vi "FormatDMAelement_6_elements.vi"(8 "valid in":bool, 10 "factor":u16, 11 "Data in":fxp<+/-,32,14>[](array[numeric])=[0.0, 0.0, 0.0, 0.0, 0.0, 0.0]) -> (0 "valid out":bool, 3 "Values":u64[](array[numeric]))   [LabVIEW 2018]
uses:
  <vilib>/rvi/FXPMathLib/FxpConvert/subVIs/nifxpmath_Convert_SimConfig.ctl
  <vilib>/fxp/LVFixedPointQuantizationPolicyTypeDef.ctl
  <vilib>/fxp/LVFixedPointOverflowPolicyTypeDef.ctl
  <vilib>/rvi/FXPMathLib/FxpConvert/simVIs/DllFxpConvertTemp_sub.vi
  <vilib>/rvi/FXPMathLib/FxpConvert/XNode/nifxpmath_Convert.xnode
  <vilib>/rvi/FXPMathLib/FxpInterpret/XNode/nifxpmath_Interpret.xnode
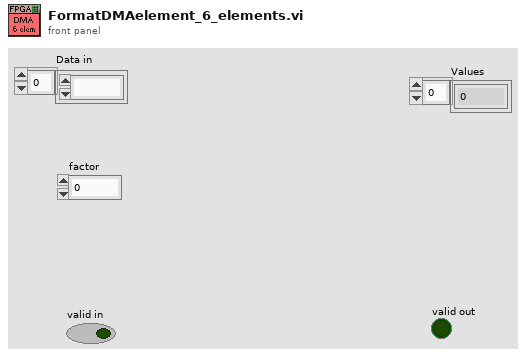
[diagram p1: front panel]
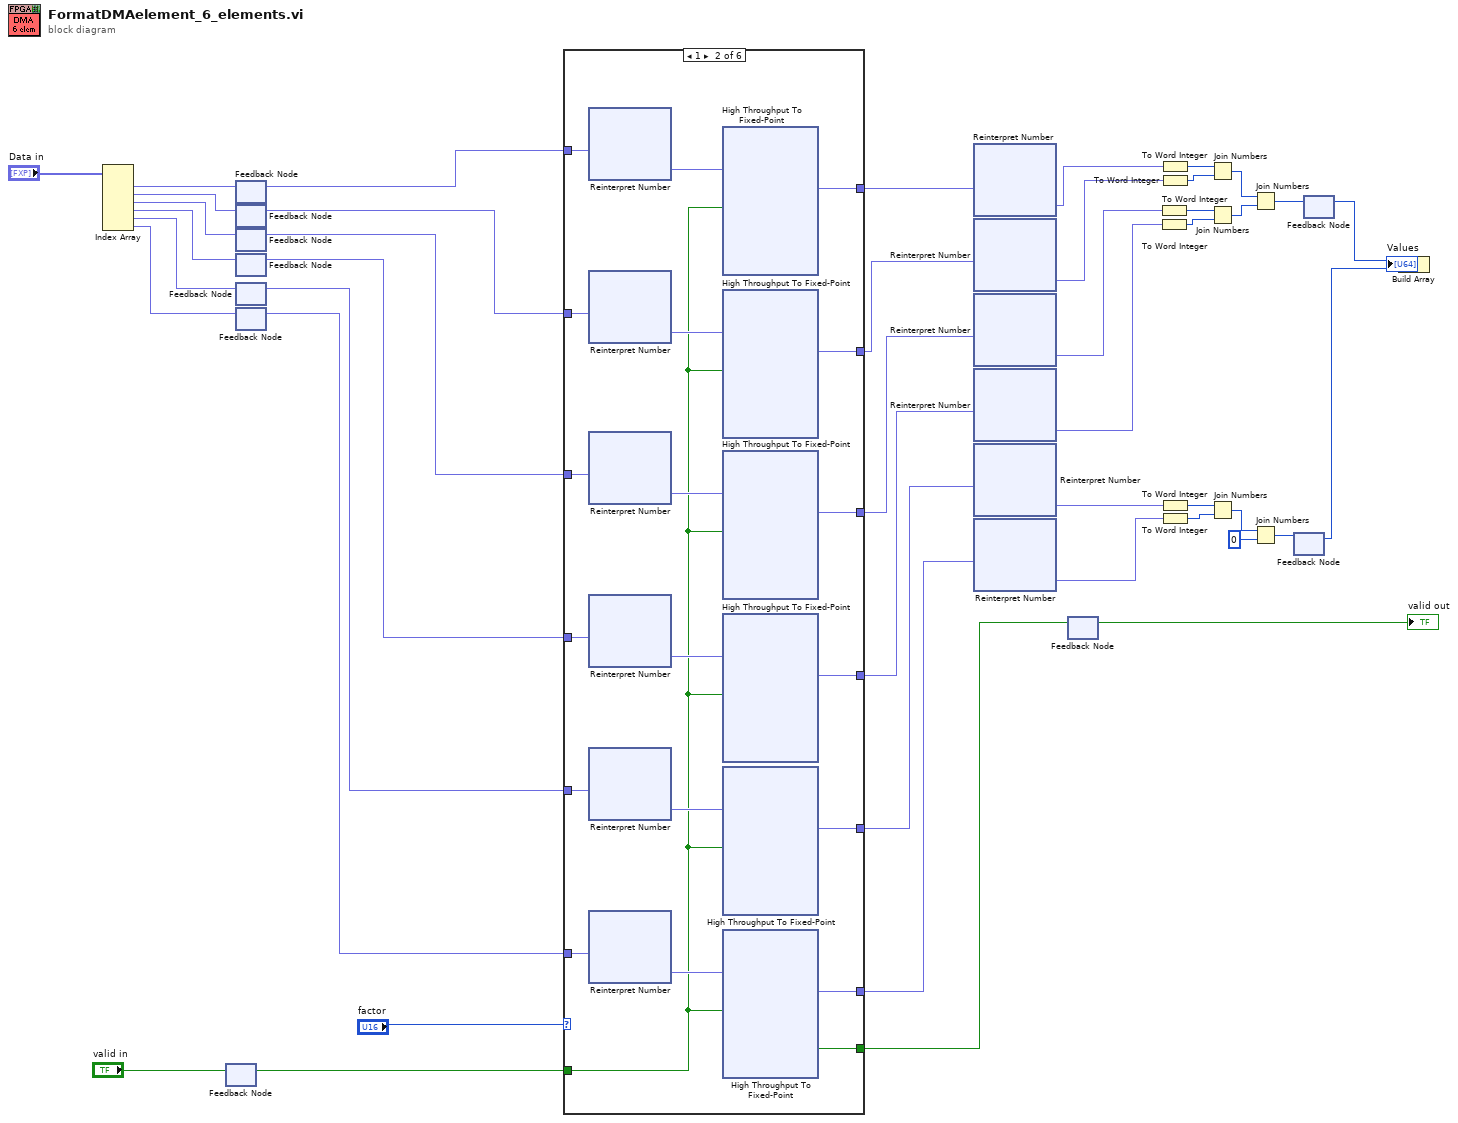
[diagram p0: block diagram]
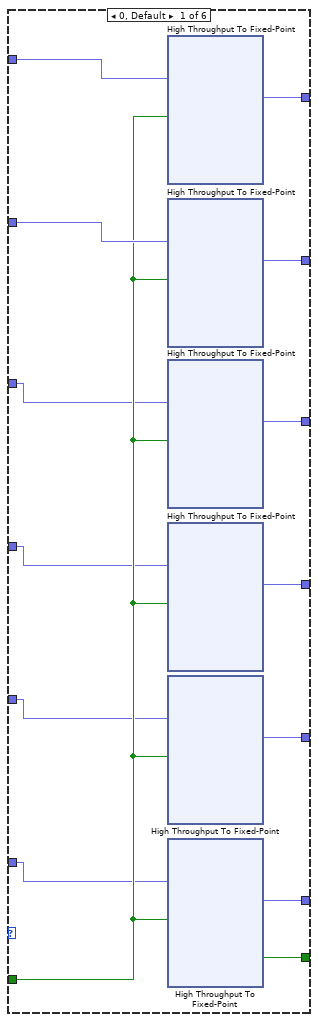
[diagram p2: hidden frame]
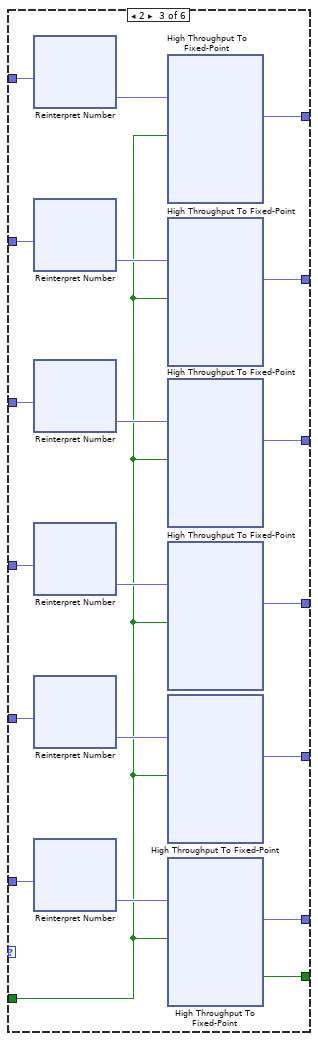
[diagram p3: hidden frame]
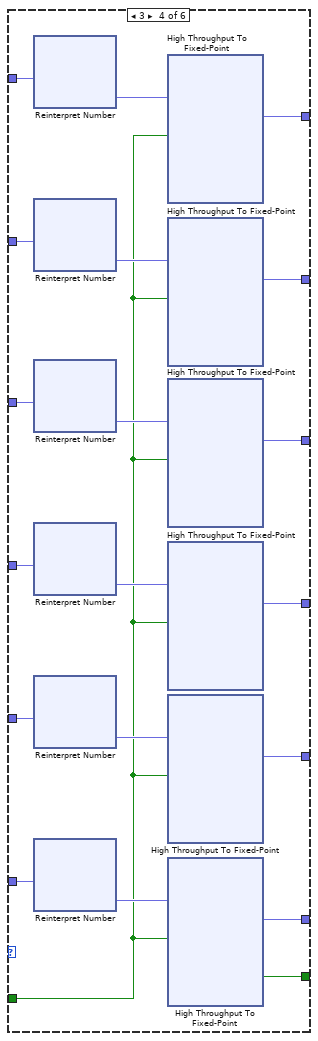
[diagram p4: hidden frame]
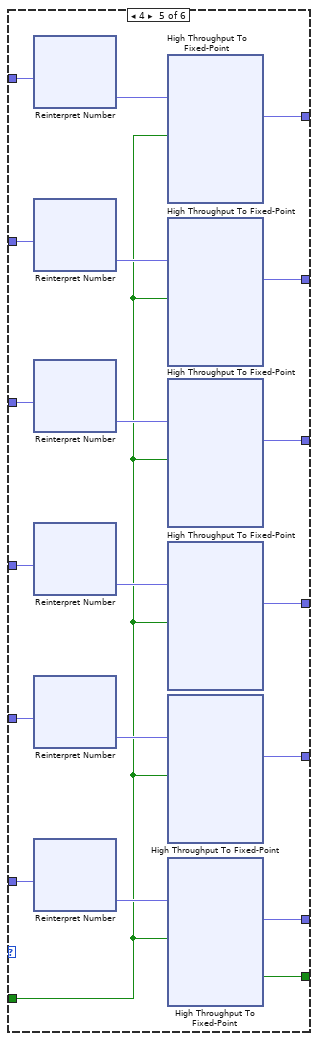
[diagram p5: hidden frame]
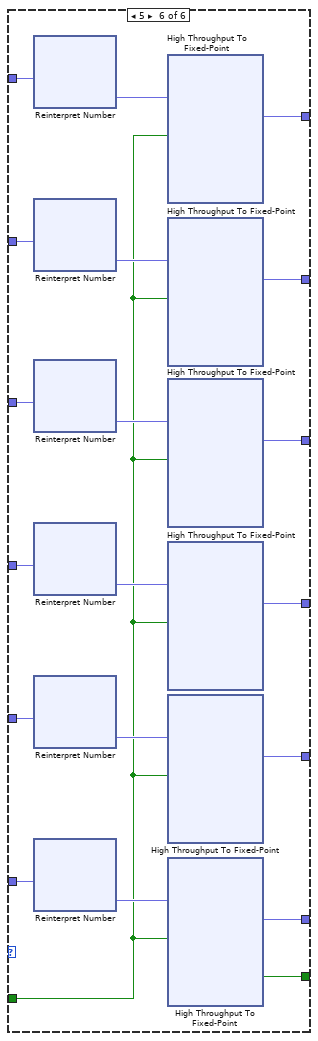
[diagram p6: hidden frame]
diagram:
  n1 = Index Array(array="Data in") -> (element #1=w43:fxp<+/-,32,14>, element #2=w42:fxp<+/-,32,14>, element #3=w41:fxp<+/-,32,14>, element #4=w40:fxp<+/-,32,14>, element #5=w33:fxp<+/-,32,14>, element #6=w32:fxp<+/-,32,14>)  [unwired: 6 in]
  n2 = feedback #1() -> (w12:bool)  [unwired: 1 in]
  n3 = feedback-in #1("valid in") -> ()
  n4 = feedback #2() -> (w15:fxp<+/-,32,14>)  [unwired: 1 in]
  n5 = feedback-in #2(w43) -> ()
  n6 = feedback #3() -> (w14:fxp<+/-,32,14>)  [unwired: 1 in]
  n7 = feedback-in #3(w42) -> ()
  n8 = feedback #4() -> (w8:fxp<+/-,32,14>)  [unwired: 1 in]
  n9 = feedback-in #4(w41) -> ()
  n10 = feedback #5() -> (w9:fxp<+/-,32,14>)  [unwired: 1 in]
  n11 = feedback-in #5(w40) -> ()
  n12 = feedback #6() -> (w10:fxp<+/-,32,14>)  [unwired: 1 in]
  n13 = feedback-in #6(w33) -> ()
  n14 = feedback #7() -> (w11:fxp<+/-,32,14>)  [unwired: 1 in]
  n15 = feedback-in #7(w32) -> ()
  n16 = case shown="1" "factor" {
    tunnel: w12 -> [w55 w205 w369 w533 w697 w861]
    tunnel: [w59 w223 w387 w551 w715 w879] -> w7
    tunnel: [w58 w222 w386 w550 w714 w878] -> w6
    tunnel: w15 -> [w57 w221 w385 w549 w713 w877]
    tunnel: w14 -> [w56 w219 w383 w547 w711 w875]
    tunnel: [w54 w212 w376 w540 w704 w868] -> w2
    tunnel: [w53 w213 w377 w541 w705 w869] -> w3
    tunnel: [w52 w207 w371 w535 w699 w863] -> w4
    tunnel: [w51 w206 w370 w534 w698 w862] -> w5
    tunnel: w11 -> [w46 w211 w375 w539 w703 w867]
    tunnel: w10 -> [w47 w210 w374 w538 w702 w866]
    tunnel: w9 -> [w48 w209 w373 w537 w701 w865]
    tunnel: w8 -> [w49 w208 w372 w536 w700 w864]
    tunnel: [w50 w204 w368 w532 w696 w860] -> w1
    frame 0, Default {
      n17 = xnode "High Throughput To Fixed-Point"("x"=w57, "input valid"=w55) -> ("y"=w59:fxp<+/-,16,14>)  [unwired: 1 in, 2 out]
      n18 = xnode "High Throughput To Fixed-Point"("x"=w56, "input valid"=w55) -> ("y"=w58:fxp<+/-,16,14>)  [unwired: 1 in, 2 out]
      n19 = xnode "High Throughput To Fixed-Point"("x"=w49, "input valid"=w55) -> ("y"=w51:fxp<+/-,16,14>)  [unwired: 1 in, 2 out]
      n20 = xnode "High Throughput To Fixed-Point"("x"=w48, "input valid"=w55) -> ("y"=w52:fxp<+/-,16,14>)  [unwired: 1 in, 2 out]
      n21 = xnode "High Throughput To Fixed-Point"("x"=w47, "input valid"=w55) -> ("y"=w53:fxp<+/-,16,14>)  [unwired: 1 in, 2 out]
      n22 = xnode "High Throughput To Fixed-Point"("x"=w46, "input valid"=w55) -> ("y"=w54:fxp<+/-,16,14>, "output valid"=w50:bool)  [unwired: 1 in, 1 out]
    }
    frame 1 {
      n23 = xnode "Reinterpret Number"("x"=w221) -> ("y"=w220:fxp<+/-,32,15>)
      n24 = xnode "Reinterpret Number"("x"=w219) -> ("y"=w218:fxp<+/-,32,15>)
      n25 = xnode "Reinterpret Number"("x"=w208) -> ("y"=w216:fxp<+/-,32,15>)
      n26 = xnode "Reinterpret Number"("x"=w209) -> ("y"=w217:fxp<+/-,32,15>)
      n27 = xnode "Reinterpret Number"("x"=w210) -> ("y"=w215:fxp<+/-,32,15>)
      n28 = xnode "Reinterpret Number"("x"=w211) -> ("y"=w214:fxp<+/-,32,15>)
      n29 = xnode "High Throughput To Fixed-Point"("x"=w220, "input valid"=w205) -> ("y"=w223:fxp<+/-,16,14>)  [unwired: 1 in, 2 out]
      n30 = xnode "High Throughput To Fixed-Point"("x"=w218, "input valid"=w205) -> ("y"=w222:fxp<+/-,16,14>)  [unwired: 1 in, 2 out]
      n31 = xnode "High Throughput To Fixed-Point"("x"=w216, "input valid"=w205) -> ("y"=w206:fxp<+/-,16,14>)  [unwired: 1 in, 2 out]
      n32 = xnode "High Throughput To Fixed-Point"("x"=w217, "input valid"=w205) -> ("y"=w207:fxp<+/-,16,14>)  [unwired: 1 in, 2 out]
      n33 = xnode "High Throughput To Fixed-Point"("x"=w215, "input valid"=w205) -> ("y"=w213:fxp<+/-,16,14>)  [unwired: 1 in, 2 out]
      n34 = xnode "High Throughput To Fixed-Point"("x"=w214, "input valid"=w205) -> ("y"=w212:fxp<+/-,16,14>, "output valid"=w204:bool)  [unwired: 1 in, 1 out]
    }
    frame 2 {
      n35 = xnode "Reinterpret Number"("x"=w385) -> ("y"=w384:fxp<+/-,32,16>)
      n36 = xnode "Reinterpret Number"("x"=w383) -> ("y"=w382:fxp<+/-,32,16>)
      n37 = xnode "Reinterpret Number"("x"=w372) -> ("y"=w380:fxp<+/-,32,16>)
      n38 = xnode "Reinterpret Number"("x"=w373) -> ("y"=w381:fxp<+/-,32,16>)
      n39 = xnode "Reinterpret Number"("x"=w374) -> ("y"=w379:fxp<+/-,32,16>)
      n40 = xnode "Reinterpret Number"("x"=w375) -> ("y"=w378:fxp<+/-,32,16>)
      n41 = xnode "High Throughput To Fixed-Point"("x"=w384, "input valid"=w369) -> ("y"=w387:fxp<+/-,16,14>)  [unwired: 1 in, 2 out]
      n42 = xnode "High Throughput To Fixed-Point"("x"=w382, "input valid"=w369) -> ("y"=w386:fxp<+/-,16,14>)  [unwired: 1 in, 2 out]
      n43 = xnode "High Throughput To Fixed-Point"("x"=w380, "input valid"=w369) -> ("y"=w370:fxp<+/-,16,14>)  [unwired: 1 in, 2 out]
      n44 = xnode "High Throughput To Fixed-Point"("x"=w381, "input valid"=w369) -> ("y"=w371:fxp<+/-,16,14>)  [unwired: 1 in, 2 out]
      n45 = xnode "High Throughput To Fixed-Point"("x"=w379, "input valid"=w369) -> ("y"=w377:fxp<+/-,16,14>)  [unwired: 1 in, 2 out]
      n46 = xnode "High Throughput To Fixed-Point"("x"=w378, "input valid"=w369) -> ("y"=w376:fxp<+/-,16,14>, "output valid"=w368:bool)  [unwired: 1 in, 1 out]
    }
    frame 3 {
      n47 = xnode "Reinterpret Number"("x"=w549) -> ("y"=w548:fxp<+/-,32,17>)
      n48 = xnode "Reinterpret Number"("x"=w547) -> ("y"=w546:fxp<+/-,32,17>)
      n49 = xnode "Reinterpret Number"("x"=w536) -> ("y"=w544:fxp<+/-,32,17>)
      n50 = xnode "Reinterpret Number"("x"=w537) -> ("y"=w545:fxp<+/-,32,17>)
      n51 = xnode "Reinterpret Number"("x"=w538) -> ("y"=w543:fxp<+/-,32,17>)
      n52 = xnode "Reinterpret Number"("x"=w539) -> ("y"=w542:fxp<+/-,32,17>)
      n53 = xnode "High Throughput To Fixed-Point"("x"=w548, "input valid"=w533) -> ("y"=w551:fxp<+/-,16,14>)  [unwired: 1 in, 2 out]
      n54 = xnode "High Throughput To Fixed-Point"("x"=w546, "input valid"=w533) -> ("y"=w550:fxp<+/-,16,14>)  [unwired: 1 in, 2 out]
      n55 = xnode "High Throughput To Fixed-Point"("x"=w544, "input valid"=w533) -> ("y"=w534:fxp<+/-,16,14>)  [unwired: 1 in, 2 out]
      n56 = xnode "High Throughput To Fixed-Point"("x"=w545, "input valid"=w533) -> ("y"=w535:fxp<+/-,16,14>)  [unwired: 1 in, 2 out]
      n57 = xnode "High Throughput To Fixed-Point"("x"=w543, "input valid"=w533) -> ("y"=w541:fxp<+/-,16,14>)  [unwired: 1 in, 2 out]
      n58 = xnode "High Throughput To Fixed-Point"("x"=w542, "input valid"=w533) -> ("y"=w540:fxp<+/-,16,14>, "output valid"=w532:bool)  [unwired: 1 in, 1 out]
    }
    frame 4 {
      n59 = xnode "Reinterpret Number"("x"=w713) -> ("y"=w712:fxp<+/-,32,18>)
      n60 = xnode "Reinterpret Number"("x"=w711) -> ("y"=w710:fxp<+/-,32,18>)
      n61 = xnode "Reinterpret Number"("x"=w700) -> ("y"=w708:fxp<+/-,32,18>)
      n62 = xnode "Reinterpret Number"("x"=w701) -> ("y"=w709:fxp<+/-,32,18>)
      n63 = xnode "Reinterpret Number"("x"=w702) -> ("y"=w707:fxp<+/-,32,18>)
      n64 = xnode "Reinterpret Number"("x"=w703) -> ("y"=w706:fxp<+/-,32,18>)
      n65 = xnode "High Throughput To Fixed-Point"("x"=w712, "input valid"=w697) -> ("y"=w715:fxp<+/-,16,14>)  [unwired: 1 in, 2 out]
      n66 = xnode "High Throughput To Fixed-Point"("x"=w710, "input valid"=w697) -> ("y"=w714:fxp<+/-,16,14>)  [unwired: 1 in, 2 out]
      n67 = xnode "High Throughput To Fixed-Point"("x"=w708, "input valid"=w697) -> ("y"=w698:fxp<+/-,16,14>)  [unwired: 1 in, 2 out]
      n68 = xnode "High Throughput To Fixed-Point"("x"=w709, "input valid"=w697) -> ("y"=w699:fxp<+/-,16,14>)  [unwired: 1 in, 2 out]
      n69 = xnode "High Throughput To Fixed-Point"("x"=w707, "input valid"=w697) -> ("y"=w705:fxp<+/-,16,14>)  [unwired: 1 in, 2 out]
      n70 = xnode "High Throughput To Fixed-Point"("x"=w706, "input valid"=w697) -> ("y"=w704:fxp<+/-,16,14>, "output valid"=w696:bool)  [unwired: 1 in, 1 out]
    }
    frame 5 {
      n71 = xnode "Reinterpret Number"("x"=w877) -> ("y"=w876:fxp<+/-,32,19>)
      n72 = xnode "Reinterpret Number"("x"=w875) -> ("y"=w874:fxp<+/-,32,19>)
      n73 = xnode "Reinterpret Number"("x"=w864) -> ("y"=w872:fxp<+/-,32,19>)
      n74 = xnode "Reinterpret Number"("x"=w865) -> ("y"=w873:fxp<+/-,32,19>)
      n75 = xnode "Reinterpret Number"("x"=w866) -> ("y"=w871:fxp<+/-,32,19>)
      n76 = xnode "Reinterpret Number"("x"=w867) -> ("y"=w870:fxp<+/-,32,19>)
      n77 = xnode "High Throughput To Fixed-Point"("x"=w876, "input valid"=w861) -> ("y"=w879:fxp<+/-,16,14>)  [unwired: 1 in, 2 out]
      n78 = xnode "High Throughput To Fixed-Point"("x"=w874, "input valid"=w861) -> ("y"=w878:fxp<+/-,16,14>)  [unwired: 1 in, 2 out]
      n79 = xnode "High Throughput To Fixed-Point"("x"=w872, "input valid"=w861) -> ("y"=w862:fxp<+/-,16,14>)  [unwired: 1 in, 2 out]
      n80 = xnode "High Throughput To Fixed-Point"("x"=w873, "input valid"=w861) -> ("y"=w863:fxp<+/-,16,14>)  [unwired: 1 in, 2 out]
      n81 = xnode "High Throughput To Fixed-Point"("x"=w871, "input valid"=w861) -> ("y"=w869:fxp<+/-,16,14>)  [unwired: 1 in, 2 out]
      n82 = xnode "High Throughput To Fixed-Point"("x"=w870, "input valid"=w861) -> ("y"=w868:fxp<+/-,16,14>, "output valid"=w860:bool)  [unwired: 1 in, 1 out]
    }
  }
  n83 = xnode "Reinterpret Number"("x"=w7) -> ("y"=w22:fxp<+/-,16,16>)
  n84 = xnode "Reinterpret Number"("x"=w6) -> ("y"=w21:fxp<+/-,16,16>)
  n85 = xnode "Reinterpret Number"("x"=w5) -> ("y"=w20:fxp<+/-,16,16>)
  n86 = xnode "Reinterpret Number"("x"=w4) -> ("y"=w19:fxp<+/-,16,16>)
  n87 = xnode "Reinterpret Number"("x"=w3) -> ("y"=w18:fxp<+/-,16,16>)
  n88 = xnode "Reinterpret Number"("x"=w2) -> ("y"=w17:fxp<+/-,16,16>)
  n89 = feedback #8() -> (→"valid out":bool)  [unwired: 1 in]
  n90 = feedback-in #8(w1) -> ()
  n91 = To Word Integer(number=w20) -> (16bit integer=w37:i16)
  n92 = To Word Integer(number=w19) -> (16bit integer=w36:i16)
  n93 = To Word Integer(number=w22) -> (16bit integer=w38:i16)
  n94 = To Word Integer(number=w21) -> (16bit integer=w39:i16)
  n95 = To Word Integer(number=w18) -> (16bit integer=w30:i16)
  n96 = To Word Integer(number=w17) -> (16bit integer=w29:i16)
  n97 = Join Numbers(hi=w38, lo=w39) -> ((hi.lo)=w35:u32)
  n98 = Join Numbers(hi=w37, lo=w36) -> ((hi.lo)=w34:u32)
  n99 = Join Numbers(hi=w30, lo=w29) -> ((hi.lo)=w31:u32)
  n100 = Join Numbers(hi=w35, lo=w34) -> ((hi.lo)=w27:u64)
  n101 = Join Numbers(hi=w31, lo=u32 0) -> ((hi.lo)=w26:u64)
  n102 = feedback #9() -> (w25:u64)  [unwired: 1 in]
  n103 = feedback-in #9(w26) -> ()
  n104 = feedback #10() -> (w24:u64)  [unwired: 1 in]
  n105 = feedback-in #10(w27) -> ()
  n106 = Build Array(w24, w25) -> (→"Values":u64[])
